vi "Configure DC Bias.vi"(7 "Enable DC Bias (F: Disable)":bool, 8 "error in (no error)":errorcluster, 9 "Bias Port (0: LF Output port)":i32(ring) items=["LF Output port", "Port 1"], 10 "DC Bias Voltage (0 V)":dbl, 11 "VISA resource name":refnum<visa-resource-name>) -> (0 "error out":errorcluster, 3 "VISA resource name out":refnum<visa-resource-name>)   [LabVIEW 2018, in "Agilent ENA Series.lvlib"]
doc: "Configures the DC Bias settings.\n\n<B>Note:</B>This VI is only available for E5061B."
uses:
  Agilent ENA Series.lvlib
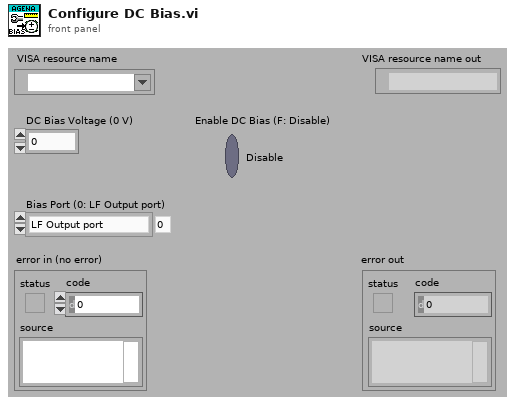
[diagram p1: front panel]
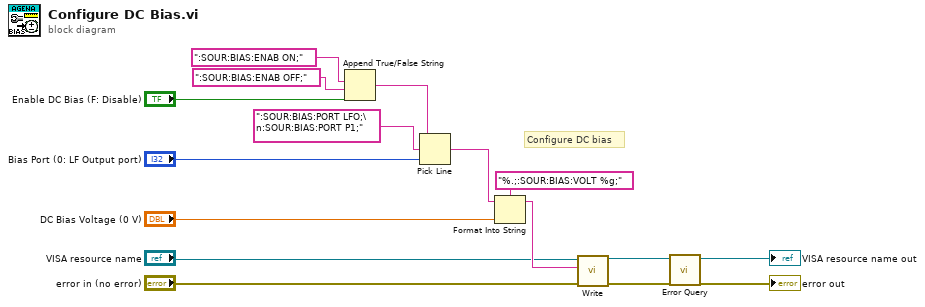
[diagram p0: block diagram]
diagram:
  # "Configure DC bias"
  n1 = Append True/False String(1:"Enable DC Bias (F: Disable)", 2:":SOUR:BIAS:ENAB OFF;", 3:":SOUR:BIAS:ENAB ON;") -> (0:w11:string)  [unwired: 1 out]
  n2 = Pick Line(string ("")=w11, multi-line string=":SOUR:BIAS:PORT LFO;\n:SOUR:BIAS:PORT P1;", line index="Bias Port (0: LF Output port)") -> (output string=w10:string)
  n3 = Format Into String(format string="%.;:SOUR:BIAS:VOLT %g;", initial string=w10, "DC Bias Voltage (0 V)") -> (resulting string=w3:string)  [unwired: 1 in, 1 out]
  n4 = call "Write.vi"("error in (no error)"="error in (no error)", "String ()"=w3, "VISA resource name"="VISA resource name") -> ("error out"=w4:errorcluster, "VISA resource name out"=w5:refnum<visa-resource-name>)  [unwired: 6 in, 1 out]
  n5 = call "Error Query.vi"("error in (no error)"=w4, "VISA resource name"=w5) -> ("error out"=→"error out":errorcluster, "VISA resource name out"=→"VISA resource name out":refnum<visa-resource-name>)  [unwired: 8 out]
